vi "Add Header Auth.vi"(8 "error in":errorcluster, 10 "Api Token":string="8y3UfvlU-s_u9u_oxA6shSxOW3EspqNUnOF1NvG3HuRk3uhql6GwvIuXxEX0eFPkzaJQUr8iPPkS1eW6XzXgRw==", 11 "client handle in":T1) -> (0 "error out":errorcluster, 3 "client handle out":T1)   [LabVIEW 2020, in "InfluxDB v2 Client.lvlib"]
doc: "Creates the header for authentification"
uses:
  InfluxDB v2 Client.lvlib
  <vilib>/httpClient/ClientHandle.ctl
  <vilib>/httpClient/LabVIEWHTTPClient.lvlib
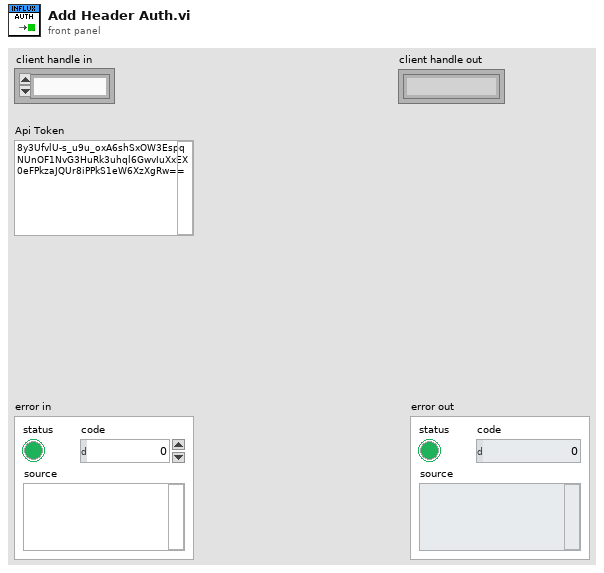
[diagram p1: front panel]
types:
  T1 = typedef "LabVIEWHTTPClient.lvlib/ClientHandle.ctl" = refnum<k1>
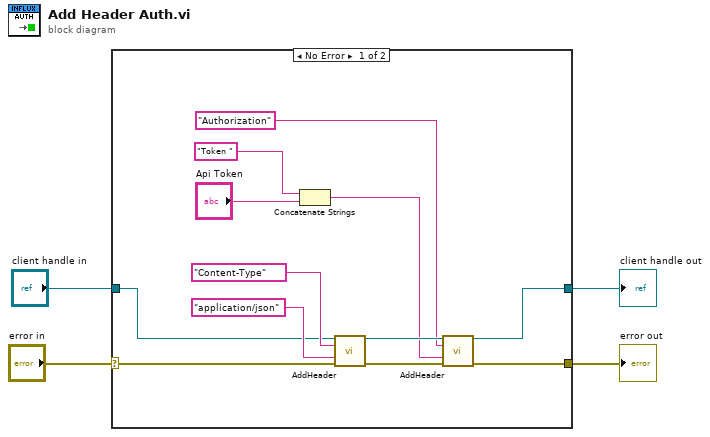
[diagram p0: block diagram]
diagram:
  n1 = case shown="No Error" "error in" {
    selector: "error in" -> [w9 w17]
    tunnel: [w8 w17] -> w3
    tunnel: "client handle in" -> [w6 w18]
    tunnel: [w5 w18] -> w1
    frame No Error {
      n2 = Concatenate Strings("Token ", "Api Token") -> (w10:string)
      n3 = call <vilib>:"AddHeader.vi"("client handle"=w6, "header"="Content-Type", "value"="application/json", "error in (no error)"=w9) -> ("client handle out"=w14:T1, "error out"=w13:errorcluster)  [unwired: 10 in]
      n4 = call <vilib>:"AddHeader.vi"("client handle"=w14, "header"="Authorization", "value"=w10, "error in (no error)"=w13) -> ("client handle out"=w5:T1, "error out"=w8:errorcluster)  [unwired: 10 in]
    }
    frame Error {
    }
  }
  "client handle out" <- w1
  "error out" <- w3
